vi "Sound Stereo Correlation.vi"() -> ()   [LabVIEW 2017]
uses:
  <vilib>/Analysis/NI_AALBase.lvlib
panel:
  out "м/с":dbl=3360.00000000037
  out "Глаз2":dbl(knob)=-2.083333333333104e-05 scale=0.0002..-0.0002
  out "Глаз1":dbl(knob)=-2.083333333333104e-05 scale=0.0002..-0.0002
  in  "База (м)":dbl=0.07
  out "Осциллограммы":waveform(dbl)[](graph)=[{"t0"=timestamp(3606705447.3232203 s since 1904-01-01), "dt"=1.0416666666666666e-05, "Y"=array[19200 elements]}, {"t0"=timestamp(3606705447.3232203 s since 1904-01-01), "dt"=1.0416666666666666e-05, "Y"=array[19200 elements]}]
  in  "Duration (s)":dbl=0.3
  in  "stop":bool
  out "Корреляционная функция":cluster{dbl, "dt":dbl, "Rxy":dbl[]}(graph)={-0.19998958333333333, "dt"=1.0416666666666666e-05, "Rxy"=array[38399 elements]}
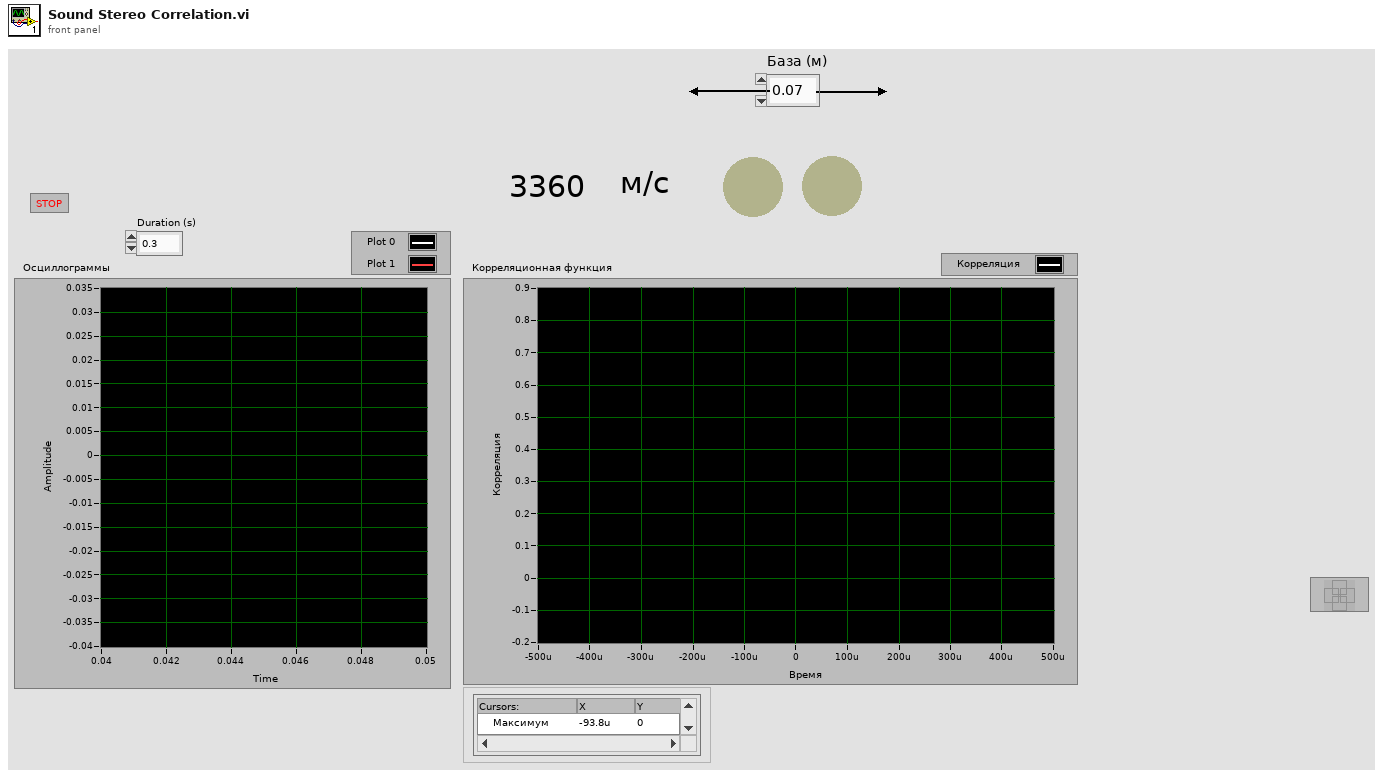
[diagram p1: front panel]
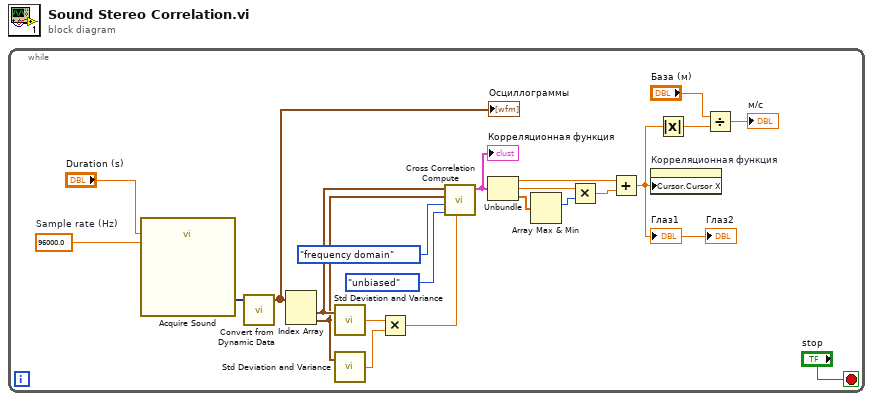
[diagram p0: block diagram]
diagram:
  n1 = while {
    stop <- "stop" stop-if-true
    w19 = 96000.0  # Sample rate (Hz)
    n2 = call "Acquire Sound"("Duration (s)"="Duration (s)", "Sample rate (Hz)"=w19) -> ("Data"=w22:dynamicdata)  [unwired: 16 in, 1 out]
    n3 = call "Convert from Dynamic Data"("Dynamic Data Type"=w22) -> ("Array of Waveform"=w16:waveform(dbl)[])  [unwired: 3 in]
    "Осциллограммы" <- w16
    n4 = Index Array(array=w16) -> (element #1=w15:waveform(dbl), element #2=w14:waveform(dbl))  [unwired: 2 in]
    n5 = call <vilib>:"Std Deviation and Variance.vi"("X"=w15) -> ("standard deviation"=w10:dbl)  [unwired: 1 in, 2 out]
    n6 = call <vilib>:"Std Deviation and Variance.vi"("X"=w14) -> ("standard deviation"=w9:dbl)  [unwired: 1 in, 2 out]
    n7 = Multiply(x=w10, y=w9) -> (x*y=w11:dbl)
    n8 = call "Cross Correlation Compute.vi"("Scale"=w11, "normalization"=enum32{"none", "unbiased", "biased"}."unbiased", "algorithm"=enum32{"direct", "frequency domain"}."frequency domain", "Waveform 2"=w14, "Waveform 1"=w15) -> ("Cross Correlation"=w8:cluster{dbl, "dt":dbl, dbl[]})  [unwired: 6 in]
    "Корреляционная функция" <- w8
    n9 = Unbundle(w8) -> (w6:dbl, "dt"=w4:dbl, w7:dbl[])
    n10 = Array Max & Min(array=w7) -> (max index (indices)=w5:i32)  [unwired: 3 out]
    n11 = Multiply(x=w4, y=w5) -> (x*y=w3:dbl)
    n12 = Add(x=w6, y=w3) -> (x+y=w1:dbl)
    "Глаз1" <- w1
    "Глаз2" <- w1
    n13 = property on="Корреляционная функция" class="WFGraph (strict)"("Cursor.Cursor X"=w1) -> ()  [unwired: 2 in, 2 out]
    n14 = Absolute Value(x=w1) -> (abs(x)=w2:dbl)
    n15 = Divide(x="База (м)", y=w2) -> (x/y=→"м/с":dbl)
  }
